vi "Configuration Tool Main.vi"() -> ()   [LabVIEW 2015, in "Configuration Tool.lvlib"]
doc: "This is the main VI for the configuration editor."
uses:
  Configuration Tool.lvlib
  Controls/StateCluster.ctl
  <vilib>/NI/Configuration Framework/Repository/NISE_CEF_Repository.lvclass
  <vilib>/NI/Configuration Framework/Node/NodeRef.ctl
  <vilib>/NI/Configuration Framework/Node/NISE_CEF_Node.lvclass
  <vilib>/NI/Configuration Framework/Node/StandardEvents.ctl
  <vilib>/NI/Configuration Framework/Node/UserEventRef.ctl
  <vilib>/NI/Configuration Framework/Controls/EventCluster.ctl
  <vilib>/NI/Configuration Framework/Node/NodeChangeEvent.ctl
  <vilib>/NI/Configuration Framework/Node/CacheState.ctl
  <vilib>/NI/Configuration Framework/Node/RefreshUIEvent.ctl
  <vilib>/NI/Configuration Framework/Node/StopEvent.ctl
  <vilib>/NI/Configuration Framework/glyph manager/glyph manager.ctl
  <vilib>/picture/picture.llb/imagedata.ctl
  Controls/AddMessage.ctl
  Controls/MoveMessage.ctl
  <vilib>/Utility/error.llb/DialogType.ctl
  Classes/cRIO/cRIO.lvclass
  Classes/cRIO Repo/cRIORepo.lvclass
  <vilib>/Utility/sysdir.llb/System Directory Type.ctl
  <vilib>/NI/AMC/Read Termination Message.vi
  <vilib>/NI/AMC/Create Single Message.vi
  <vilib>/NI/AMC/Update Message Routing Info.vi
  <vilib>/NI/AMC/Send Message.vi
  <vilib>/NI/AMC/Globals.vi
  <vilib>/NI/AMC/AMC.lvlib
  <vilib>/NI/Configuration Framework/NISE_CEF_TreeControl.lvlib
  <vilib>/NI/Configuration Framework/glyph manager/glyph manager.lvlib
panel:
  in  "View":string(tree)
  in  "Exit":bool
  # "Configurator"
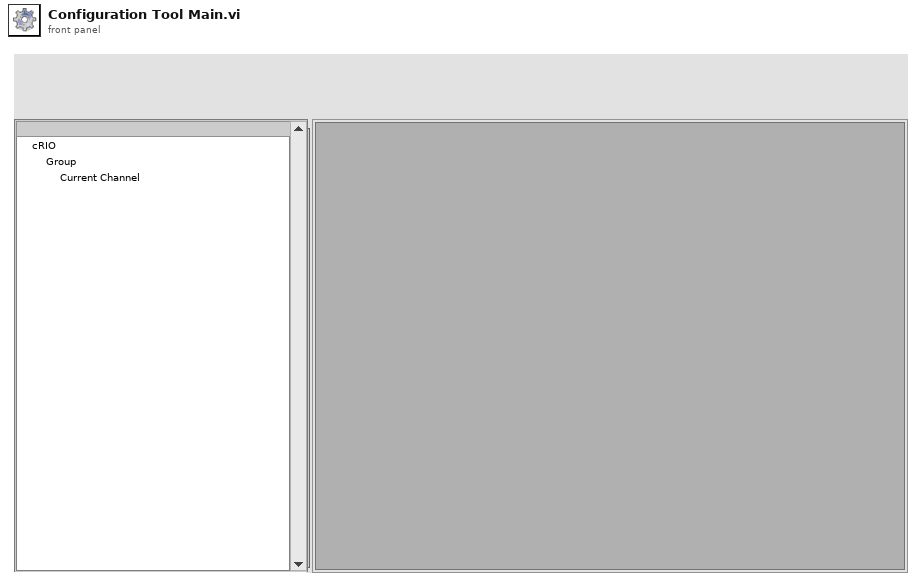
[diagram p1: front panel]
types:
  T1 = typedef "Configuration Tool.lvlib/StateCluster.ctl" = cluster{"repository":refnum<class "NISE_CEF_Repository.lvclass">, "root":T2, "unsaved changes":bool, "current path":path, "standard events":T3, "classes path":path, "glyph manager":T9}
  T2 = typedef "NISE_CEF_Node.lvclass/NodeRef.ctl" = refnum<data-value>
  T3 = typedef "NISE_CEF_Node.lvclass/StandardEvents.ctl" = cluster{"user event":T4, "node change":T5, "cache state":T6, "refresh UI":T7, "stop event":T8}
  T4 = typedef "NISE_CEF_Node.lvclass/UserEventRef.ctl" = refnum<user-event>
  T5 = typedef "NISE_CEF_Node.lvclass/NodeChangeEvent.ctl" = refnum<user-event>
  T6 = typedef "NISE_CEF_Node.lvclass/CacheState.ctl" = refnum<user-event>
  T7 = typedef "NISE_CEF_Node.lvclass/RefreshUIEvent.ctl" = refnum<user-event>
  T8 = typedef "NISE_CEF_Node.lvclass/StopEvent.ctl" = refnum<user-event>
  T9 = typedef "glyph manager.lvlib/glyph manager.ctl" = cluster{"search paths":path[], "glyph map":variant, "base glyphs":T10[], "desired overlays":string[]}
  T10 = typedef "imagedata.ctl" = cluster{"image type":i32, "image depth":i32, "image":u8[], "mask":u8[], "colors":u32[], "Rectangle":cluster{"left":i16, "top":i16, "right":i16, "bottom":i16}}
  T11 = typedef "AMC.lvlib/Message Queue.ctl" = refnum<queue>
  T12 = typedef "Configuration Tool.lvlib/AddMessage.ctl" = cluster{"node type":string, "to add to":string}
  T13 = typedef "Configuration Tool.lvlib/MoveMessage.ctl" = cluster{"node ref":T2, "new parent":T2}
  T14 = typedef "Configuration Tool.lvlib/FilePaths.ctl" = cluster{"glyphs":path, "classes":path}
  T15 = typedef "DialogType.ctl" = u16
  T16 = typedef "System Directory Type.ctl" = i32
  T17 = typedef "NISE_CEF_Node.lvclass/Summary.ctl" = cluster{"ID":string, "parent ID":string, "node type":string, "text":string, "additional text":string, "glyph":string, "depth":i32, "glyph overlay":string}
  T18 = typedef "LVPoint32TypeDef.ctl" = cluster{"Horizontal":i32, "Vertical":i32}
  T19 = cluster{"data name":string, "drag data":variant}[]
  T20 = typedef "NISE_CEF_Node.lvclass/NodeMenuOptions.ctl" = cluster{"removable":bool, "movable":bool, "duplicate":bool}
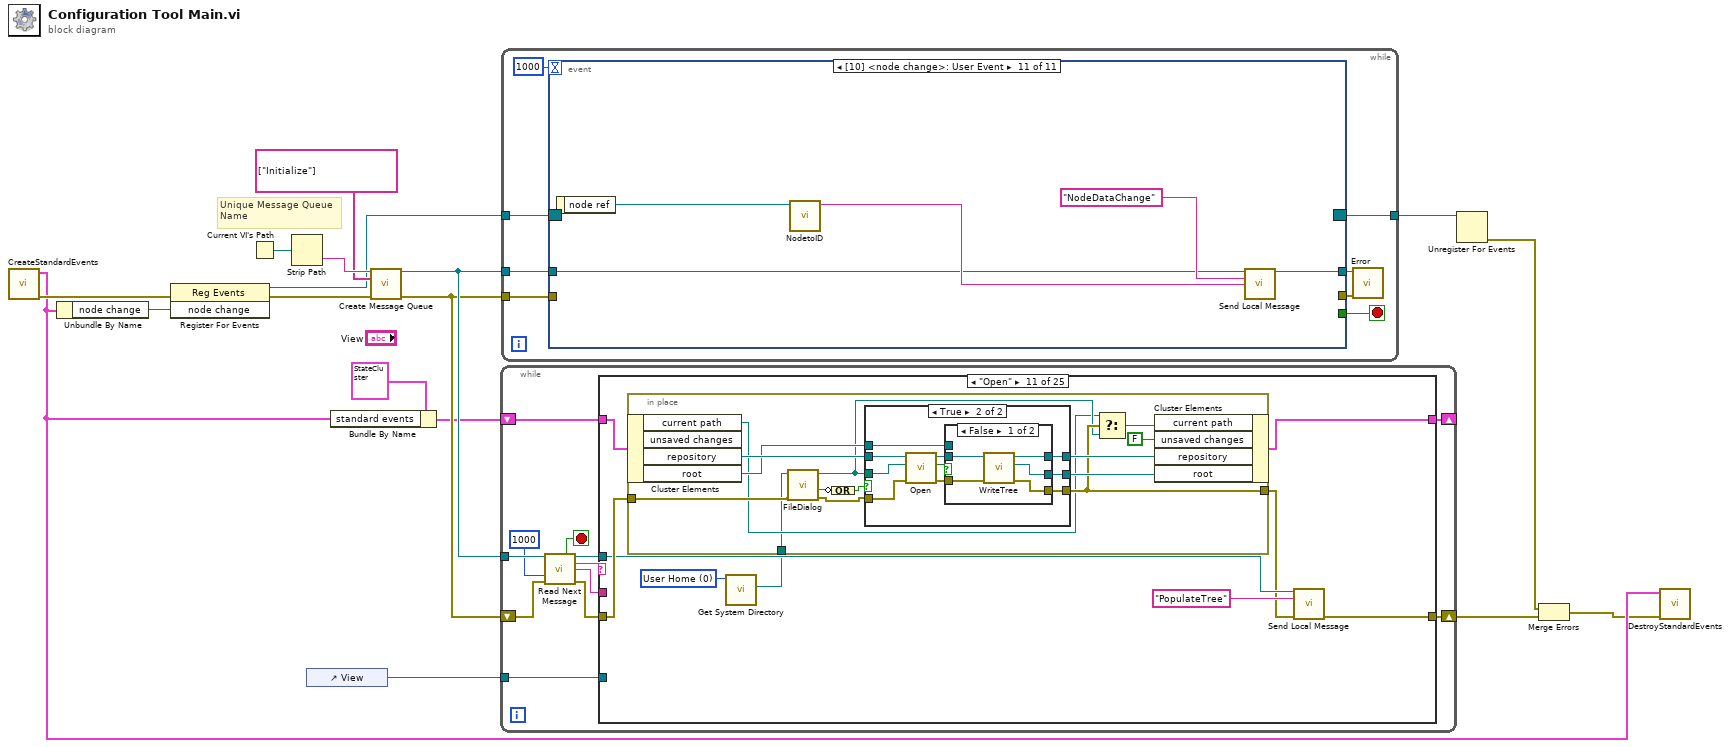
[diagram p0: block diagram]
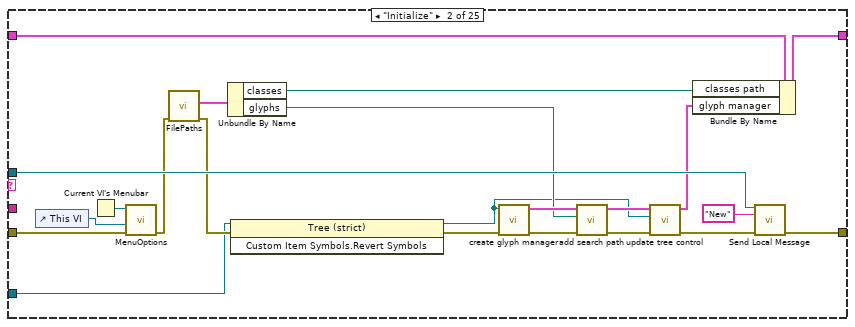
[diagram p3: hidden frame]
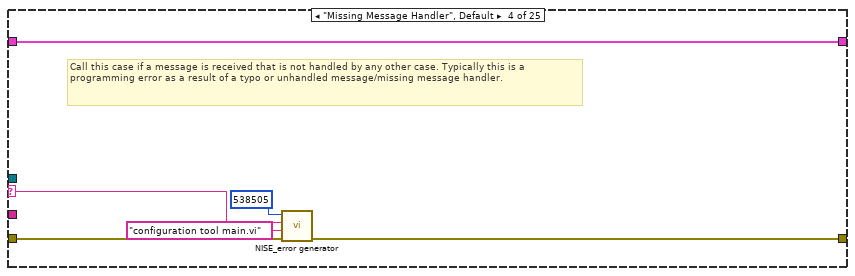
[diagram p5: hidden frame]
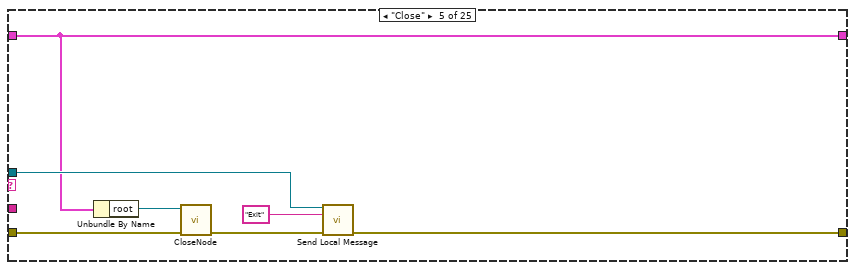
[diagram p6: hidden frame]
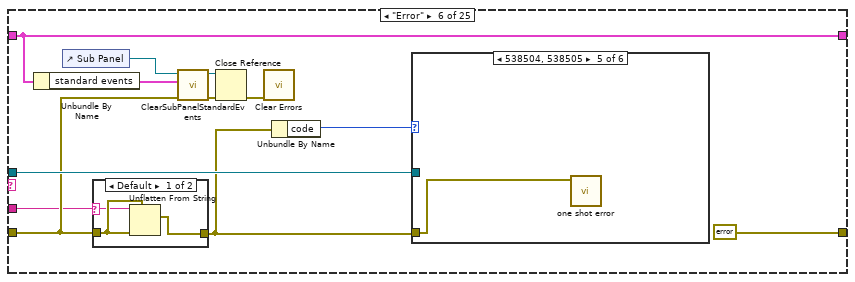
[diagram p7: hidden frame]
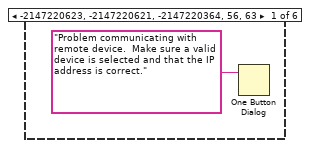
[diagram p9: hidden frame]
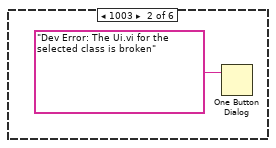
[diagram p10: hidden frame]
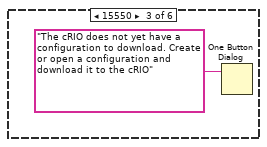
[diagram p11: hidden frame]
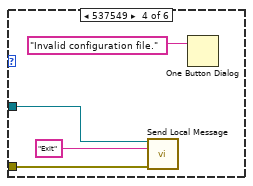
[diagram p12: hidden frame]
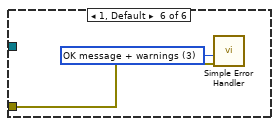
[diagram p13: hidden frame]
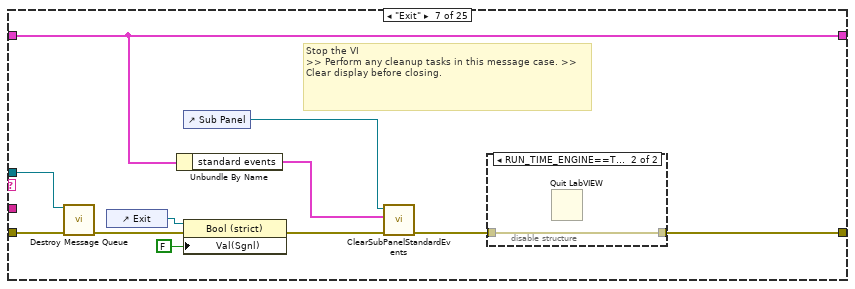
[diagram p14: hidden frame]
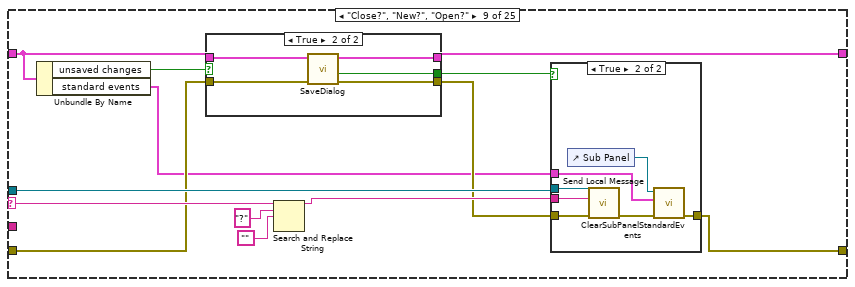
[diagram p17: hidden frame]
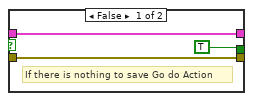
[diagram p18: hidden frame]
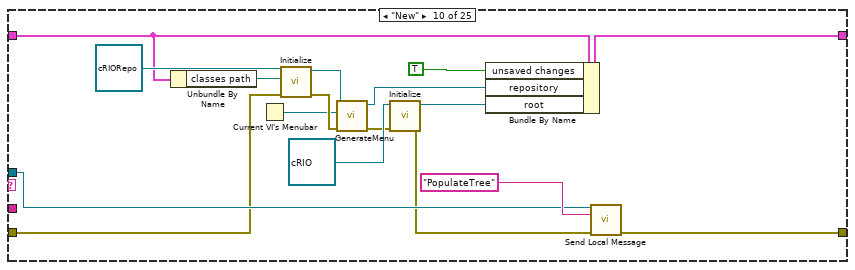
[diagram p20: hidden frame]
diagram:
  # "Unique Message Queue Name"
  n1 = call <vilib>:"CreateStandardEvents.vi"() -> ("error out"=w12:errorcluster, "standard events"=w6:T3)  [unwired: 10 in]
  n2 = Unbundle By Name(w6) -> ("node change"=w11:T5)
  n3 = register-events(error in=w12, w11) -> (reference out=w5:refnum<event-registration>, error out=w10:errorcluster)  [unwired: 1 in]
  n4 = Current VI's Path() -> (path=w16:path)
  n5 = Strip Path(path=w16) -> (name=w17:string)  [unwired: 1 out]
  n6 = control-ref of="View"() -> (w4:refnum<vi>)
  n7 = Bundle By Name(cluster=T1 {"repository"=refnum, "root"=refnum, "unsaved changes"=FALSE, "current path"=path "", "standard events"={"user event"=refnum, "node change"=refnum, "cache state"=refnum, "refresh UI"=refnum, "stop event"=refnum}, "classes path"=path "", "glyph manager"={"search paths"=[], "glyph map"=variant, "base glyphs"=[], "desired overlays"=[]}}, "standard events"=w6) -> (w8:T1)
  n8 = call <vilib>:"Create Message Queue.vi"("message queue name"=w17, "initial message names"=string[] ["Initialize"], "error in"=w10) -> ("message queue out"=w14:T11, "error out"=w13:errorcluster)  [unwired: 11 in]
  n9 = while "Message Processor" {
    shift-right: [w25] -> w7
    shift-left: w13 -> [w24]
    tunnel: w14 -> [w23]
    shift-right: [w21] -> _
    shift-left: w8 -> [w20]
    tunnel: w4 -> [w18]
    stop <- w29 stop-if-true
    n10 = call <vilib>:"Read Next Message.vi"("message queue in"=w23, "timeout (1 ms)"=1000, "error in"=w24) -> ("exit process?"=w29:bool, "message queue out"=w19:T11, "message name"=w28:string, "message value"=w27:string, "error out"=w26:errorcluster)  [unwired: 5 in, 3 out]
    n11 = case shown="\"Open\"" w28 {
      selector: w28 -> [_ _ _ w57 _ _ _ _ w118 _ _ _ _ _ _ _ _ w318 _ _ _ _ _ _ _]
      tunnel: w27 -> [_ _ _ _ _ w70 _ _ _ _ _ _ _ w236 _ w279 w296 w316 w368 w392 _ _ w432 w452 w459]
      tunnel: w26 -> [w31 w53 w55 w60 w63 w73 w105 w109 w111 w144 w162 w202 w228 w243 w256 w271 w295 w321 w370 w391 w413 w422 w431 w450 w460]
      tunnel: [w31 w49 w55 w58 w67 errorcluster {"status"=FALSE, "code"=0, "source"=""} ("error out") w97 w109 w122 w154 w158 w206 w230 w240 w256 w273 w299 w324 w372 w388 w407 w418 w428 w445 w458] -> w25
      tunnel: [w30 w45 w54 w61 w65 w77 w96 w108 w113 w152 w163 w209 w229 w237 w255 w265 w292 w325 w371 w393 w404 w421 w426 w453 w455] -> w21
      tunnel: w20 -> [w30 w46 w54 w61 w65 w77 w96 w108 w114 w147 w164 w204 w227 w238 w255 w269 w293 w325 w363 w393 w416 w421 w426 w453 w461]
      tunnel: w19 -> [_ w48 _ _ w66 w80 w104 _ w121 w153 w160 w205 _ w239 _ _ _ w319 _ _ _ _ w427 w444 w457]
      tunnel: w18 -> [_ w32 _ _ _ _ _ _ _ _ _ _ _ _ _ w266 w288 w313 w365 w386 w405 _ _ _ _]
      frame "------------Generic Operations------------" {
        # "Dummy case to add a seperation in the Case Structure menu"
      }
      frame "Initialize" {
        n12 = control-ref of="This VI"() -> (w52:refnum<vi>)
        n13 = Current VI's Menubar() -> (w51:refnum<k9>)
        n14 = call "MenuOptions.vi"("error in"=w53, "VI ref"=w52, "menu ref in"=w51) -> ("error out"=w44:errorcluster)  [unwired: 7 in, 1 out]
        n15 = call "FilePaths.vi"("error in"=w44) -> ("error out"=w35:errorcluster, "paths"=w47:T14)  [unwired: 9 in]
        n16 = Unbundle By Name(w47) -> ("classes"=w43:path, "glyphs"=w37:path)
        n17 = invoke class="Tree (strict)" method="Custom Item Symbols.Revert Symbols"(reference=w32, error in=w35) -> (reference out=w33:refnum<vi>, error out=w34:errorcluster)  [unwired: 1 in, 1 out]
        n18 = call <vilib>:"create glyph manager.vi"("error in"=w34, "tree ref (for default symbols)"=w33) -> ("error out"=w42:errorcluster, "glyph manager"=w41:T9)  [unwired: 8 in]
        n19 = call <vilib>:"add search path.vi"("error in"=w42, "search path"=w37, "glyph manager in"=w41) -> ("error out"=w40:errorcluster, "glyph manager out"=w39:T9)  [unwired: 7 in]
        n20 = call <vilib>:"update tree control.vi"("error in"=w40, "tree reference"=w33, "glyph manager in"=w39) -> ("error out"=w38:errorcluster, "glyph manager out"=w36:T9)  [unwired: 7 in]
        n21 = Bundle By Name(cluster=w46, "classes path"=w43, "glyph manager"=w36) -> (w45:T1)
        n22 = call <vilib>:"Send Local Message.vi"("message queue in"=w48, "message name"="New" ("Message Name"), "error in"=w38) -> ("error out"=w49:errorcluster)  [unwired: 10 in, 2 out]
      }
      frame "", "Idle" {
      }
      frame "Missing Message Handler", Default {
        # "Call this case if a message is received that is not handled by any other case. Typically this is a programming error as a result of a typo or unhandled message/missing message handler."
        n23 = call <vilib>:"NISE_error generator.vi"("error in"=w60, "source"="configuration tool main.vi", "append error message"=w57, "error code (0)"=538505) -> ("error out"=w58:errorcluster)  [unwired: 5 in]
      }
      frame "Close" {
        n24 = Unbundle By Name(w65) -> ("root"=w64:T2)
        n25 = call <vilib>:"CloseNode.vi"("error in"=w63, "node ref"=w64) -> ("error out"=w62:errorcluster)  [unwired: 9 in]
        n26 = call <vilib>:"Send Local Message.vi"("message queue in"=w66, "message name"="Exit", "error in"=w62) -> ("error out"=w67:errorcluster)  [unwired: 10 in, 2 out]
      }
      frame "Error" {
        n27 = Unbundle By Name(w77) -> ("standard events"=w69:T3)
        n28 = control-ref of="Sub Panel"() -> (w76:refnum<vi>)
        n29 = case shown="Default" w70 {
          selector: w70 -> [w82 _]
          tunnel: w73 -> [w83 w84]
          tunnel: [w81 w84] -> w72
          frame Default {
            n30 = Unflatten From String(type=w83, binary string=w82, error in (no error)=w83) -> (value=w81:errorcluster)  [unwired: 2 in, 2 out]
          }
          frame "" {
          }
        }
        n31 = call <vilib>:"ClearSubPanelStandardEvents.vi"("error in"=w73, "standard events"=w69, "sub panel ref in"=w76) -> ("error out"=w75:errorcluster, "sub panel ref out"=w74:refnum<vi>)  [unwired: 7 in]
        n32 = Close Reference(reference=w74, error in (no error)=w75) -> (error out=w71:errorcluster)
        n33 = call <vilib>:"Clear Errors.vi"("error in (no error)"=w71) -> ()  [unwired: 5 in, 2 out]
        n34 = Unbundle By Name(w72) -> ("code"=w78:i32)
        n35 = case shown="538504, 538505" w78 {
          tunnel: w80 -> [_ _ _ w90 _ _]
          tunnel: w72 -> [_ _ _ w89 w92 w94]
          frame -2147220623, -2147220621, -2147220364, 56, 63 {
            n36 = One Button Dialog(message="Problem communicating with remote device.  Make sure a valid device is selected and that the IP address is correct.") -> ()  [unwired: 1 in, 1 out]
          }
          frame 1003 {
            n37 = One Button Dialog(message="Dev Error: The Ui.vi for the selected class is broken") -> ()  [unwired: 1 in, 1 out]
          }
          frame 15550 {
            n38 = One Button Dialog(message="The cRIO does not yet have a configuration to download. Create or open a configuration and download it to the cRIO") -> ()  [unwired: 1 in, 1 out]
          }
          frame 537549 {
            n39 = call <vilib>:"Send Local Message.vi"("message queue in"=w90, "message name"="Exit", "error in"=w89) -> ()  [unwired: 10 in, 3 out]
            n40 = One Button Dialog(message="Invalid configuration file.") -> ()  [unwired: 1 in, 1 out]
          }
          frame 538504, 538505 {
            n41 = call <vilib>:"one shot error.vi"("error in"=w92) -> ()  [unwired: 11 in]
          }
          frame 1, Default {
            w93 = T15 3 items=["no dialog", "OK message", "continue or stop message", "OK message + warnings", "continue/stop + warnings"] ("type of dialog (OK msg:1)")
            n42 = call <vilib>:"Simple Error Handler.vi"("type of dialog (OK msg:1)"=w93, "error in (no error)"=w94) -> ()  [unwired: 8 out]
          }
        }
      }
      frame "Exit" {
        # "Stop the VI                                                                             >> Perform any cleanup tasks in this message case. >> Clear display before closing."
        n43 = call <vilib>:"Destroy Message Queue.vi"("message queue in"=w104, "error in"=w105) -> ("error out"=w101:errorcluster)  [unwired: 11 in, 2 out]
        n44 = control-ref of="Exit"() -> (w103:refnum<vi>)
        n45 = Unbundle By Name(w96) -> ("standard events"=w95:T3)
        n46 = control-ref of="Sub Panel"() -> (w100:refnum<vi>)
        n47 = property class="Bool (strict)"(reference=w103, error in=w101, "Val(Sgnl)"=FALSE ("Exit")) -> (error out=w99:errorcluster)  [unwired: 1 out]
        n48 = call <vilib>:"ClearSubPanelStandardEvents.vi"("error in"=w99, "standard events"=w95, "sub panel ref in"=w100) -> ("error out"=w98:errorcluster)  [unwired: 7 in, 1 out]
        n49 = disable-structure shown="RUN_TIME_ENGINE==True" {
          disable-tunnel: [w106 w107] -> w97
          disable-tunnel: w98 -> [w106 w107]
          frame condition #0 (active) {
          }
          frame condition #1 {
            n50 = Quit LabVIEW() -> ()  [unwired: 1 in]
          }
        }
      }
      frame "------------Menu Operations--------------" {
        # "Dummy case to add a seperation in the Case Structure menu"
      }
      frame "Close?", "New?", "Open?" {
        n51 = Unbundle By Name(w114) -> ("unsaved changes"=w116:bool, "standard events"=w110:T3)
        n52 = case shown="True" w116 {
          tunnel: [TRUE ("SaveFlag") w130] -> w115
          tunnel: w114 -> [w124 w129]
          tunnel: [w124 w128] -> w113
          tunnel: w111 -> [w123 w127]
          tunnel: [w123 w126] -> w112
          frame False {
            # "If there is nothing to save Go do Action"
          }
          frame True {
            n53 = call "SaveDialog.vi"("error in"=w127, "state in"=w129) -> ("error out"=w126:errorcluster, "new"=w130:bool, "state out"=w128:T1)  [unwired: 7 in]
          }
        }
        n54 = Search and Replace String(input string=w118, search string="?", replace string="") -> (result string=w117:string)  [unwired: 5 in, 3 out]
        n55 = case shown="True" w115 {
          tunnel: w112 -> [w131 w138]
          tunnel: [w131 w134] -> w122
          tunnel: w121 -> [_ w137]
          tunnel: w117 -> [_ w136]
          tunnel: w110 -> [_ w132]
          frame False {
          }
          frame True {
            n56 = control-ref of="Sub Panel"() -> (w133:refnum<vi>)
            n57 = call <vilib>:"Send Local Message.vi"("message queue in"=w137, "message name"=w136, "error in"=w138) -> ("error out"=w135:errorcluster)  [unwired: 10 in, 2 out]
            n58 = call <vilib>:"ClearSubPanelStandardEvents.vi"("error in"=w135, "standard events"=w132, "sub panel ref in"=w133) -> ("error out"=w134:errorcluster)  [unwired: 7 in, 1 out]
          }
        }
      }
      frame "New" {
        n59 = Unbundle By Name(w147) -> ("classes path"=w146:path)
        n60 = Current VI's Menubar() -> (w139:refnum<k9>)
        n61 = call-dynamic "Initialize.vi"("error in"=w144, "path"=w146, "repository in"=refnum<class "cRIORepo.lvclass"> refnum ("cRIORepo.lvclass")) -> ("error out"=w143:errorcluster, "repository out"=w141:refnum<class "cRIORepo.lvclass">)  [unwired: 7 in]
        n62 = call-dynamic "GenerateMenu.vi"("error in"=w143, "menu ref in"=w139, "NISE_CEF_Repository in"=w141) -> ("error out"=w142:errorcluster, "NISE_CEF_Repository out"=w140:refnum<class "cRIORepo.lvclass">)  [unwired: 6 in, 1 out]
        n63 = call-dynamic "Initialize.vi"("error in"=w142, "cRIO in"=refnum<class "cRIO.lvclass"> refnum ("cRIO.lvclass")) -> ("error out"=w145:errorcluster, "data value reference"=w149:T2)  [unwired: 7 in, 1 out]
        n64 = Bundle By Name(cluster=w147, "unsaved changes"=TRUE ("SaveFlag"), "repository"=w140, "root"=w149) -> (w152:T1)
        n65 = call <vilib>:"Send Local Message.vi"("message queue in"=w153, "message name"="PopulateTree", "error in"=w145) -> ("error out"=w154:errorcluster)  [unwired: 10 in, 2 out]
      }
      frame "Open" {
        w157 = T16 0 items=["User Home"=0, "User Desktop"=1, "User Documents"=2, "User Application Data"=3, "User Preferences"=4, "User Temporary"=5, "Public Documents"=6, "Public Application Data"=7, "Public Preferences"=8, "Public Cache"=13, "System Core Libraries"=9, "System Installed Libraries"=10, "Application Files"=11, "Boot Volume Root"=12] ("system directory type")
        n66 = call <vilib>:"Get System Directory.vi"("system directory type"=w157) -> ("system directory"=w156:path)  [unwired: 10 in]
        n67 = in-place {
          in-place-border: w162 -> [w170]
          in-place-border: [w169] -> w159
          in-place-border: w156 -> [w165]
          n68 = in-place-cluster #1(w164) -> ("current path"=w167:path, "repository"=w178:refnum<class "NISE_CEF_Repository.lvclass">, "root"=w174:T2)  [unwired: 1 out]
          n69 = call "FileDialog.vi"("error in"=w170, "start path"=w165) -> ("error out"=w171:errorcluster, "cancelled"=w172:bool, "selected path"=w168:path)  [unwired: 7 in]
          n70 = Compound Arithmetic op=OR(invert w172) -> (w173:bool)
          n71 = case shown="True" w173 {
            tunnel: w178 -> [w179 w191]
            tunnel: [w179 w189] -> w176
            tunnel: [w180 w187] -> w169
            tunnel: [w181 w186] -> w175
            tunnel: w168 -> [_ w184]
            tunnel: w171 -> [w180 w183]
            tunnel: w174 -> [w181 w182]
            frame False {
            }
            frame True {
              n72 = call-dynamic "Open.vi"("error in"=w183, "file path"=w184, "repository in"=w191) -> ("error out"=w188:errorcluster, "invalid?"=w185:bool, "repository out"=w190:refnum<class "NISE_CEF_Repository.lvclass">)  [unwired: 6 in]
              n73 = case shown="False" w185 {
                tunnel: w190 -> [w196 w199]
                tunnel: [w195 w199] -> w189
                tunnel: w188 -> [w194 w198]
                tunnel: [w193 w198] -> w187
                tunnel: [w192 w197] -> w186
                tunnel: w182 -> [_ w197]
                frame False {
                  n74 = call-dynamic "WriteTree.vi"("error in"=w194, "repository in"=w196) -> ("error out"=w193:errorcluster, "root"=w192:T2, "repository out"=w195:refnum<class "NISE_CEF_Repository.lvclass">)  [unwired: 7 in]
                }
                frame True {
                }
              }
            }
          }
          n75 = Select(t=w167, s=w169, f=w168) -> (s? t:f=w166:path)
          n76 = in-place-cluster #1("current path"=w166, "unsaved changes"=FALSE ("SaveFlag"), "repository"=w176, "root"=w175) -> (w163:T1)
        }
        n77 = call <vilib>:"Send Local Message.vi"("message queue in"=w160, "message name"="PopulateTree", "error in"=w159) -> ("error out"=w158:errorcluster)  [unwired: 10 in, 2 out]
      }
      frame "Save" {
        n78 = in-place {
          in-place-border: w202 -> [w213]
          in-place-border: [w212] -> w201
          in-place-border: [w210] -> w200
          n79 = in-place-cluster #2(w204) -> ("current path"=w211:path, "root"=w214:T2, "repository"=w216:refnum<class "NISE_CEF_Repository.lvclass">)
          n80 = Empty String/Path?(string/path=w211) -> (empty?=w210:bool)
          n81 = call-dynamic "ReadTree.vi"("error in"=w213, "root"=w214, "repository in"=w216) -> ("error out"=w212:errorcluster, "repository out"=w215:refnum<class "NISE_CEF_Repository.lvclass">)  [unwired: 7 in]
          n82 = in-place-cluster #2("current path"=w211, "root"=w214, "repository"=w215) -> (w203:T1)
        }
        n83 = case shown="True" w200 {
          tunnel: w203 -> [w220 w222]
          tunnel: [w219 w221] -> w209
          tunnel: [w218 w223] -> w207
          tunnel: w201 -> [w217 w224]
          frame False {
            n84 = call "Save.vi"("error in"=w217, "state in"=w220) -> ("error out"=w218:errorcluster, "state out"=w219:T1)  [unwired: 8 in]
          }
          frame True {
            # "Empty path use Dialog"
            n85 = call "SaveAs.vi"("error in"=w224, "state in"=w222) -> ("error out"=w223:errorcluster, "state out"=w221:T1)  [unwired: 7 in, 1 out]
          }
        }
        n86 = call <vilib>:"Send Local Message.vi"("message queue in"=w205, "message name"="PopulateTree", "error in"=w207) -> ("error out"=w206:errorcluster)  [unwired: 10 in, 2 out]
      }
      frame "SaveAs" {
        n87 = in-place {
          in-place-border: w228 -> [w232]
          in-place-border: [w231] -> w226
          n88 = in-place-cluster #3(w227) -> ("root"=w233:T2, "repository"=w235:refnum<class "NISE_CEF_Repository.lvclass">)
          n89 = call-dynamic "ReadTree.vi"("error in"=w232, "root"=w233, "repository in"=w235) -> ("error out"=w231:errorcluster, "repository out"=w234:refnum<class "NISE_CEF_Repository.lvclass">)  [unwired: 7 in]
          n90 = in-place-cluster #3("root"=w233, "repository"=w234) -> (w225:T1)
        }
        n91 = call "SaveAs.vi"("error in"=w226, "state in"=w225) -> ("error out"=w230:errorcluster, "state out"=w229:T1)  [unwired: 7 in, 1 out]
      }
      frame "Custom View" {
        n92 = in-place {
          in-place-border: w243 -> [w254]
          in-place-border: [w253] -> w241
          in-place-border: w236 -> [w244]
          n93 = in-place-cluster #4(w238) -> ("repository"=w248:refnum<class "NISE_CEF_Repository.lvclass">, "root"=w247:T2)
          n94 = call-dynamic "ReadTree.vi"("error in"=w254, "root"=w247, "repository in"=w248) -> ("error out"=w251:errorcluster, "repository out"=w250:refnum<class "NISE_CEF_Repository.lvclass">)  [unwired: 7 in]
          n95 = call-dynamic "CustomView.vi"("error in"=w251, "view name"=w244, "repository in"=w250) -> ("error out"=w252:errorcluster, "repository out"=w249:refnum<class "NISE_CEF_Repository.lvclass">)  [unwired: 7 in]
          n96 = call-dynamic "WriteTree.vi"("error in"=w252, "repository in"=w249) -> ("error out"=w253:errorcluster, "root"=w245:T2, "repository out"=w246:refnum<class "NISE_CEF_Repository.lvclass">)  [unwired: 7 in]
          n97 = in-place-cluster #4("repository"=w246, "root"=w245) -> (w237:T1)
        }
        n98 = call <vilib>:"Send Local Message.vi"("message queue in"=w239, "message name"="PopulateTree", "error in"=w241) -> ("error out"=w240:errorcluster)  [unwired: 10 in, 2 out]
      }
      frame "-------TreeControl Operations-----------" {
        # "Dummy case to add a seperation in the Case Structure menu"
      }
      frame "AddNode" {
        n99 = Unflatten From String(type=T12 {"node type"="", "to add to"=""} ("input cluster"), binary string=w279) -> (value=w277:T12)  [unwired: 3 in, 2 out]
        n100 = Unbundle By Name(w277) -> ("to add to"=w275:string, "node type"=w268:string)
        n101 = in-place {
          in-place-border: w271 -> [w285]
          in-place-border: [w284] -> w270
          in-place-border: w268 -> [w283]
          in-place-border: [w282] -> w267
          n102 = in-place-cluster #5(w269) -> ("repository"=w287:refnum<class "NISE_CEF_Repository.lvclass">)
          n103 = call-dynamic "GetClassPath.vi"("error in"=w285, "class name"=w283, "Repository in"=w287) -> ("error out"=w284:errorcluster, "class path"=w282:path, "Repository out"=w286:refnum<class "NISE_CEF_Repository.lvclass">)  [unwired: 6 in]
          n104 = in-place-cluster #5("repository"=w286) -> (w262:T1)
        }
        n105 = Unbundle By Name(w262) -> ("glyph manager"=w261:T9)
        n106 = call <vilib>:"Get LV Class Default Value.vi"("error in (no error)"=w270, "class path"=w267) -> ("error out"=w280:errorcluster, "object"=w281:refnum<class>)  [unwired: 8 in]
        n107 = To More Specific Class(target class=refnum<class "NISE_CEF_Node.lvclass"> refnum ("Node.lvclass"), reference=w281, error in=w280) -> (specific class reference=w263:refnum<class "NISE_CEF_Node.lvclass">, error out=w264:errorcluster)
        n108 = call-dynamic "AddGlyphtoGManager.vi"("error in"=w264, "glyph manager"=w261, "NISE_CEF_Node in"=w263) -> ("error out"=w259:errorcluster, "glyph manager out"=w260:T9, "NISE_CEF_Node out"=w258:refnum<class "NISE_CEF_Node.lvclass">)  [unwired: 6 in]
        n109 = call <vilib>:"AddNode.vi"("error in"=w259, "node in"=w258, "parent node ID"=w275) -> ("error out"=w274:errorcluster, "summary"=w272:T17[])  [unwired: 7 in]
        n110 = call <vilib>:"PopulateTreeSumaryWithGlyphManager.vi"("error in"=w274, "glyph manager"=w260, "summary"=w272, "tree ref in"=w266) -> ("error out"=w273:errorcluster, "glyph manager out"=w257:T9)  [unwired: 6 in]
        n111 = Bundle By Name(cluster=w262, "glyph manager"=w257) -> (w265:T1)
      }
      frame "Duplicate" {
        n112 = call <vilib>:"IDtoNode.vi"("error in"=w295, "ID"=w296) -> ("error out"=w297:errorcluster, "invalid Id"=w294:bool, "node ref"=w298:T2)  [unwired: 7 in]
        n113 = Unbundle By Name(w293) -> ("glyph manager"=w290:T9)
        n114 = case shown="False" w294 {
          tunnel: [w310 w312] -> w299
          tunnel: w298 -> [w309 _]
          tunnel: w297 -> [w306 w312]
          tunnel: w290 -> [w302 w311]
          tunnel: [w301 w311] -> w289
          tunnel: w288 -> [w300 _]
          frame False {
            n115 = call <vilib>:"DuplicateNode.vi"("same parent?"=TRUE ("s"), "error in"=w306, "node ref in"=w309) -> ("error out"=w307:errorcluster, "new node ref"=w308:T2)  [unwired: 7 in]
            n116 = call <vilib>:"Summary.vi"("error in"=w307, "node self ref"=w308) -> ("error out"=w304:errorcluster, "summary"=w303:T17[])  [unwired: 8 in]
            n117 = call <vilib>:"PopulateTreeSumaryWithGlyphManager.vi"("error in"=w304, "glyph manager"=w302, "summary"=w303, "tree ref in"=w300) -> ("error out"=w310:errorcluster, "glyph manager out"=w301:T9)  [unwired: 6 in]
          }
          frame True {
          }
        }
        n118 = Bundle By Name(cluster=w293, "unsaved changes"=TRUE, "glyph manager"=w289) -> (w292:T1)
      }
      frame "CustomMenuAction" {
        n119 = Match Pattern(string=w316, regular expression=":") -> (before substring=w315:string, after substring=w314:string)  [unwired: 1 in, 2 out]
        n120 = call <vilib>:"IDtoNode.vi"("error in"=w321, "ID"=w314) -> ("error out"=w322:errorcluster, "invalid Id"=w320:bool, "node ref"=w323:T2)  [unwired: 7 in]
        n121 = case shown="False" w320 {
          tunnel: [w331 w361] -> w324
          tunnel: w323 -> [w328 _]
          tunnel: w322 -> [w334 w361]
          tunnel: w319 -> [w335 _]
          tunnel: w318 -> [_ _]
          tunnel: w315 -> [w332 _]
          tunnel: w313 -> [w329 _]
          frame False {
            n122 = in-place {
              in-place-border: w335 -> [w359]
              in-place-border: w334 -> [w357]
              in-place-border: [w356] -> w330
              in-place-border: [w355] -> w333
              in-place-border: w332 -> [w354]
              in-place-border: w329 -> [w353]
              in-place-border: [w352] -> w327
              n123 = in-place-dvr #6(w328) -> (w360:refnum<class "NISE_CEF_Node.lvclass">)  [unwired: 1 out]
              n124 = call-dynamic "MenuHandler.vi"("tree control"=w353, "main message queue"=w359, "error in"=w357, "menu string"=w354, "NISE_CEF_Node in"=w360) -> ("error out"=w356:errorcluster, "refresh tree?"=w352:bool, "Unhandled"=w355:bool, "NISE_CEF_Node out"=w358:refnum<class "NISE_CEF_Node.lvclass">)  [unwired: 3 in]
              n125 = in-place-dvr #6(w358) -> (w326:T2)  [unwired: 1 out]
            }
            n126 = case shown="False" w333 {
              tunnel: w332 -> [_ w347]
              tunnel: [w339 w348] -> w331
              tunnel: w330 -> [w337 w349]
              tunnel: w327 -> [w336 _]
              tunnel: w326 -> [w338 _]
              frame False {
                n127 = case shown="False" w336 {
                  tunnel: [w340 w343] -> w339
                  tunnel: w338 -> [_ w342]
                  tunnel: w337 -> [w340 w341]
                  frame False {
                  }
                  frame True {
                    n128 = call <vilib>:"NodetoID.vi"("error in"=w341, "node ref"=w342) -> ("error out"=w345:errorcluster, "ID"=w346:string)  [unwired: 8 in]
                    n129 = call <vilib>:"Send Local Message.vi"("message name"="NodeDataChange", "message value"=w346, "error in"=w345) -> ("error out"=w343:errorcluster)  [unwired: 10 in, 2 out]
                  }
                }
              }
              frame True {
                n130 = call <vilib>:"NISE_error generator.vi"("error in"=w349, "source"="configuration tool main.vi", "append error message"=w347, "error code (0)"=538506) -> ("error out"=w348:errorcluster)  [unwired: 5 in]
              }
            }
          }
          frame True {
          }
        }
      }
      frame "RefreshNode" {
        # "Refreshes the node in the Tree, Sets the save flag to true. This case can be called from the UIs of the nodes"
        n131 = Unbundle By Name(w363) -> ("glyph manager"=w362:T9)
        n132 = call <vilib>:"IDtoNode.vi"("error in"=w370, "ID"=w368) -> ("error out"=w369:errorcluster, "invalid Id"=w366:bool, "node ref"=w367:T2)  [unwired: 7 in]
        n133 = case shown="False" w366 {
          tunnel: [w382 w385] -> w372
          tunnel: w369 -> [w378 w385]
          tunnel: w367 -> [w377 _]
          tunnel: w365 -> [w376 _]
          tunnel: [w375 w384] -> w364
          tunnel: w362 -> [w373 w384]
          frame False {
            n134 = call <vilib>:"SummaryWithGlyphManager.vi"("error in"=w378, "glyph manager"=w373, "node self ref"=w377) -> ("error out"=w380:errorcluster, "glyph manager out"=w374:T9, "summary"=w379:T17[])  [unwired: 6 in]
            n135 = call <vilib>:"RefreshSubTreeWithGlyphManager.vi"("error in"=w380, "glyph manager"=w374, "node information"=w379, "tree ref in"=w376) -> ("error out"=w383:errorcluster, "glyph manager out"=w375:T9, "tree ref out"=w381:refnum<vi>)  [unwired: 5 in]
            n136 = Close Reference(reference=w381, error in (no error)=w383) -> (error out=w382:errorcluster)
          }
          frame True {
          }
        }
        n137 = Bundle By Name(cluster=w363, "glyph manager"=w364) -> (w371:T1)
      }
      frame "RemoveNode" {
        n138 = call <vilib>:"IDtoNode.vi"("error in"=w391, "ID"=w392) -> ("error out"=w390:errorcluster, "invalid Id"=w387:bool, "node ref"=w389:T2)  [unwired: 7 in]
        n139 = case shown="False" w387 {
          tunnel: w390 -> [w399 w400]
          tunnel: w389 -> [w398 _]
          tunnel: [w395 w400] -> w388
          tunnel: w386 -> [w394 _]
          frame False {
            n140 = call <vilib>:"RemoveNode.vi"("error in"=w399, "node"=w398) -> ("error out"=w396:errorcluster, "node ID"=w397:string)  [unwired: 8 in]
            n141 = call <vilib>:"ClearTreeNode.vi"("error in"=w396, "tag"=w397, "tree reference"=w394) -> ("error out"=w395:errorcluster)  [unwired: 8 in]
          }
          frame True {
          }
        }
      }
      frame "PopulateTree" {
        n142 = Unbundle By Name(w416) -> ("standard events"=w406:T3, "glyph manager"=w402:T9, "root"=w411:T2)
        n143 = call <vilib>:"SummaryWithGlyphManager.vi"("error in"=w413, "glyph manager"=w402, "depth"=0 ("Depth"), "node self ref"=w411) -> ("error out"=w412:errorcluster, "glyph manager out"=w401:T9, "summary"=w415:T17[])  [unwired: 5 in]
        n144 = control-ref of="This VI"() -> (w414:refnum<vi>)
        n145 = call <vilib>:"RefreshEntireTreeWithGlyphManager.vi"("calling VI in"=w414, "error in"=w412, "glyph manager"=w401, "array"=w415, "tree ref in"=w405) -> ("error out"=w408:errorcluster, "glyph manager out"=w403:T9)  [unwired: 5 in]
        n146 = control-ref of="Sub Panel"() -> (w409:refnum<vi>)
        n147 = Bundle By Name(cluster=w416, "glyph manager"=w403) -> (w404:T1)
        n148 = call <vilib>:"ClearSubPanelStandardEvents.vi"("error in"=w408, "standard events"=w406, "sub panel ref in"=w409) -> ("error out"=w407:errorcluster)  [unwired: 7 in, 1 out]
      }
      frame "CleansubPanel" {
        n149 = Unbundle By Name(w421) -> ("standard events"=w417:T3)
        n150 = control-ref of="Sub Panel"() -> (w423:refnum<vi>)
        n151 = call <vilib>:"ClearSubPanelStandardEvents.vi"("error in"=w422, "standard events"=w417, "sub panel ref in"=w423) -> ("error out"=w420:errorcluster, "sub panel ref out"=w419:refnum<vi>)  [unwired: 7 in]
        n152 = Close Reference(reference=w419, error in (no error)=w420) -> (error out=w418:errorcluster)
      }
      frame "ActivateNode" {
        n153 = Unbundle By Name(w426) -> ("standard events"=w425:T3)
        n154 = call <vilib>:"IDtoNode.vi"("error in"=w431, "ID"=w432) -> ("error out"=w424:errorcluster, "invalid Id"=w430:bool, "node ref"=w429:T2)  [unwired: 7 in]
        n155 = case shown="False" w430 {
          tunnel: w429 -> [w439 _]
          tunnel: [w440 w441] -> w428
          tunnel: w424 -> [w437 w441]
          tunnel: w427 -> [w435 _]
          tunnel: w425 -> [w433 _]
          frame False {
            n156 = control-ref of="Sub Panel"() -> (w436:refnum<vi>)
            n157 = call <vilib>:"ClearSubPanelStandardEvents.vi"("error in"=w437, "standard events"=w433, "sub panel ref in"=w436) -> ("error out"=w438:errorcluster, "sub panel ref out"=w434:refnum<vi>)  [unwired: 7 in]
            n158 = call <vilib>:"LoadNodeUIStandardEvents.vi"("user event out"=w433, "error in"=w438, "sub panel ref in"=w434, "main queue"=w435, "node"=w439) -> ("error out"=w440:errorcluster)  [unwired: 6 in]
          }
          frame True {
          }
        }
      }
      frame "Move" {
        n159 = Unflatten From String(type=T13 {"node ref"=refnum, "new parent"=refnum} ("Cluster"), binary string=w452, error in (no error)=w450) -> (value=w449:T13, error out=w448:errorcluster)  [unwired: 2 in, 1 out]
        n160 = Unbundle By Name(w449) -> ("node ref"=w443:T2, "new parent"=w442:T2)
        n161 = call <vilib>:"MoveNode.vi"("error in"=w448, "new parent"=w442, "node"=w443) -> ("error out"=w446:errorcluster)  [unwired: 8 in]
        n162 = call <vilib>:"Send Local Message.vi"("message queue in"=w444, "message name"="PopulateTree", "error in"=w446) -> ("error out"=w445:errorcluster)  [unwired: 10 in, 2 out]
      }
      frame "NodeDataChange" {
        n163 = call <vilib>:"Send Local Message.vi"("message queue in"=w457, "message name"="RefreshNode", "message value"=w459, "error in"=w460) -> ("error out"=w458:errorcluster)  [unwired: 9 in, 2 out]
        n164 = Bundle By Name(cluster=w461, "unsaved changes"=TRUE) -> (w455:T1)
      }
    }
  }
  n165 = while "User Interface Event Handler" {
    tunnel: w14 -> [w468]
    tunnel: w13 -> [w464]
    tunnel: w5 -> [w463]
    tunnel: [w462] -> w1
    stop <- w467 stop-if-true
    n166 = event shown="[10] <node change>: User Event" {
      selector: w463 -> [_ _ _ _ _ _ _ _ _ _ _]
      dyn-events: [_ _ _ _ _ _ _ _ _ _ _] -> w462
      timeout: 1000 -> [_ _ _ _ _ _ _ _ _ _ _]
      tunnel: w468 -> [w471 w479 w503 w555 w583 w590 w619 w623 w633 w639 w685]
      tunnel: [_ _ _ _ TRUE _ _ _ _ _ _] -> w467
      tunnel: [w471 w479 w500 w553 w579 w590 w616 w623 w631 w638 w686] -> w466
      tunnel: [w470 w475 w499 w552 w580 w586 w615 w620 w629 w636 _] -> w465
      tunnel: w464 -> [w470 w478 w498 w554 w581 w589 w614 w622 w630 w637 _]
      event Timeout {
        # "Timeout code can be added here for autosave or Lock Screen"
        n167 = event-data() -> ()  [unwired: 1 in, 1 out]
      }
      event "View": Shortcut Menu Activation? {
        n168 = event-data() -> ("CtlRef"=w485:refnum<vi>, "Coords"=w484:T18, "MenuRef"=w481:refnum<k9>)  [unwired: 1 in]
        n169 = invoke class="Tree (strict)" method="Point To Row Column"(reference=w485, error in=w478, "Point"=w484) -> (error out=w477:errorcluster, "Tag"=w483:string)  [unwired: 5 in, 6 out]
        n170 = call <vilib>:"IDtoNode.vi"("error in"=w477, "ID"=w483) -> ("error out"=w473:errorcluster, "invalid Id"=w480:bool, "node ref"=w482:T2)  [unwired: 7 in]
        n171 = case shown="False" w480 {
          tunnel: w482 -> [w490 _]
          tunnel: w481 -> [w489 _]
          tunnel: [w488 _] -> w476
          tunnel: [w487 _] -> w474
          tunnel: w473 -> [w486 w496]
          tunnel: [w486 w496] -> w472
          frame False {
            n172 = in-place {
              in-place-border: w489 -> [w493]
              in-place-border: [w491] -> w488
              n173 = in-place-dvr #7(w490) -> (w495:refnum<class "NISE_CEF_Node.lvclass">, w492:errorcluster)
              n174 = call-dynamic "ShortcutMenu.vi"("error in"=w492, "menu ref in"=w493, "node in"=w495) -> ("error out"=w491:errorcluster, "node out"=w494:refnum<class "NISE_CEF_Node.lvclass">)  [unwired: 6 in, 1 out]
              n175 = in-place-dvr #7(w494) -> (w487:errorcluster)  [unwired: 1 out]
            }
          }
          frame True {
          }
        }
        n176 = Merge Errors(w474, w476, w472) -> (w475:errorcluster)
        n177 = event-data() -> ()  [unwired: 2 in, 1 out]
      }
      event "View": Shortcut Menu Selection (User) {
        n178 = event-data() -> ("ItemPath"=w502:string, "CtlRef"=w506:refnum<vi>, "Coords"=w507:T18)  [unwired: 1 in]
        n179 = invoke class="Tree (strict)" method="Point To Row Column"(reference=w506, error in=w498, "Point"=w507) -> (error out=w497:errorcluster, "Tag"=w501:string)  [unwired: 5 in, 6 out]
        n180 = Match Pattern(string=w502, regular expression=":") -> (before substring=w505:string, after substring=w504:string)  [unwired: 1 in, 2 out]
        n181 = case shown="Default" w505 {
          selector: w505 -> [w509 _ _ _]
          tunnel: w504 -> [_ _ _ w534]
          tunnel: w503 -> [w516 w523 w529 w536]
          tunnel: w501 -> [w511 w521 w527 w535]
          tunnel: [w513 w520 w526 w532] -> w500
          tunnel: [w514 w519 w524 w530] -> w499
          tunnel: w497 -> [w515 w518 w525 w531]
          frame Default {
            n182 = Concatenate Strings(w509, ":" ("string"), w511) -> (w512:string)
            n183 = call <vilib>:"Send Local Message.vi"("message queue in"=w516, "message name"="CustomMenuAction" ("Message Name"), "message value"=w512, "error in"=w515) -> ("message queue out"=w513:T11, "error out"=w514:errorcluster)  [unwired: 9 in, 1 out]
          }
          frame "Remove" {
            n184 = call <vilib>:"Send Local Message.vi"("message queue in"=w523, "message name"="RemoveNode" ("Message Name"), "message value"=w521, "error in"=w518) -> ("message queue out"=w520:T11, "error out"=w519:errorcluster)  [unwired: 9 in, 1 out]
          }
          frame "Duplicate" {
            n185 = call <vilib>:"Send Local Message.vi"("message queue in"=w529, "message name"="Duplicate" ("Message Name"), "message value"=w527, "error in"=w525) -> ("message queue out"=w526:T11, "error out"=w524:errorcluster)  [unwired: 9 in, 1 out]
          }
          frame "Add" {
            n186 = Bundle By Name(cluster=T12 {"node type"="", "to add to"=""} ("input cluster"), "node type"=w534, "to add to"=w535) -> (w537:T12)
            n187 = Flatten To String(anything=w537) -> (data string=w538:string)  [unwired: 3 in, 2 out]
            n188 = call <vilib>:"Send Local Message.vi"("message queue in"=w536, "message name"="AddNode" ("Message Name"), "message value"=w538, "error in"=w531) -> ("message queue out"=w532:T11, "error out"=w530:errorcluster)  [unwired: 9 in, 1 out]
          }
        }
      }
      event "View": Drop {
        n189 = event-data() -> ("CtlRef"=w558:refnum<vi>, "Coords"=w557:T18)  [unwired: 1 in]
        n190 = invoke class="Tree (strict)" method="Point To Row Column"(reference=w558, error in=w554, "Point"=w557) -> (reference out=w556:refnum<vi>, error out=w551:errorcluster, "Tag"=w548:string)  [unwired: 5 in, 5 out]
        n191 = call <vilib>:"ValidDragDrop.vi"("error in"=w551, "drag over"=w548, "tree ref in"=w556) -> ("error out"=w543:errorcluster, "accepted"=w546:bool, "drag"=w550:string, "tree ref out"=w560:refnum<vi>)  [unwired: 5 in]
        n192 = call <vilib>:"IDtoNode.vi"("error in"=w543, "ID"=w548) -> ("error out"=w544:errorcluster, "invalid Id"=w541:bool, "node ref"=w547:T2)  [unwired: 7 in]
        n193 = call <vilib>:"IDtoNode.vi"("error in"=w544, "ID"=w550) -> ("error out"=w542:errorcluster, "invalid Id"=w540:bool, "node ref"=w549:T2)  [unwired: 7 in]
        n194 = Compound Arithmetic op=AND(w546, invert w541, invert w540) -> (w545:bool)
        n195 = case shown="True" w545 {
          tunnel: w550 -> [_ w576]
          tunnel: w560 -> [_ w578]
          tunnel: [_ TRUE] -> w559
          tunnel: w548 -> [_ w574]
          tunnel: w555 -> [w562 w573]
          tunnel: [w562 w569] -> w553
          tunnel: [w561 w568] -> w552
          tunnel: w549 -> [_ w564]
          tunnel: w547 -> [_ w563]
          tunnel: w542 -> [w561 w565]
          frame False {
          }
          frame True {
            n196 = invoke class="Tree (strict)" method="Edit Tree Items.Move Item"(reference=w578, error in=w565, "tag"=w576, "New Parent"=w574) -> (error out=w566:errorcluster)  [unwired: 3 in, 6 out]
            n197 = Bundle By Name(cluster=T13 {"node ref"=refnum, "new parent"=refnum} ("Cluster"), "new parent"=w563, "node ref"=w564) -> (w572:T13)
            n198 = Flatten To String(anything=w572, error in (no error)=w566) -> (data string=w571:string, error out=w567:errorcluster)  [unwired: 2 in, 1 out]
            n199 = call <vilib>:"Send Local Message.vi"("message queue in"=w573, "message name"="Move", "message value"=w571, "error in"=w567) -> ("message queue out"=w569:T11, "error out"=w568:errorcluster)  [unwired: 9 in, 1 out]
          }
        }
        n200 = event-data("Accepted?"=w559) -> ()  [unwired: 1 in, 1 out]
      }
      event "Exit": Value Change {
        # "Exit the application                                           >> Stop this message generator loop    Cleaning errors if the other loop stop this one"
        n201 = event-data() -> ()  [unwired: 1 in, 1 out]
        n202 = call <vilib>:"Send Local Message.vi"("message queue in"=w583, "message name"="Close", "error in"=w581) -> ("message queue out"=w579:T11, "error out"=w584:errorcluster)  [unwired: 10 in, 1 out]
        n203 = call <vilib>:"Clear Errors.vi"("error in (no error)"=w584) -> ("error out"=w580:errorcluster)  [unwired: 5 in, 1 out]
      }
      event "View": Drag Starting? {
        n204 = event-data() -> ("Data"=w596:T19, "CtlRef"=w598:refnum<vi>, "Coords"=w597:T18)  [unwired: 1 in]
        n205 = invoke class="Tree (strict)" method="Point To Row Column"(reference=w598, error in=w589, "Point"=w597) -> (error out=w588:errorcluster, "Tag"=w595:string)  [unwired: 5 in, 6 out]
        n206 = call <vilib>:"IDtoNode.vi"("error in"=w588, "ID"=w595) -> ("error out"=w587:errorcluster, "invalid Id"=w594:bool, "node ref"=w593:T2)  [unwired: 7 in]
        n207 = case shown="False" w594 {
          tunnel: w593 -> [w606 _]
          tunnel: [w603 TRUE ("Removable")] -> w591
          tunnel: w587 -> [w602 w612]
          tunnel: [w599 w612] -> w586
          frame False {
            n208 = in-place {
              in-place-border: [w609] -> w605
              in-place-border: w602 -> [w608]
              in-place-border: [w607] -> w601
              n209 = in-place-dvr #8(w606) -> (w611:refnum<class "NISE_CEF_Node.lvclass">)  [unwired: 1 out]
              n210 = call-dynamic "EditOptions.vi"("error in"=w608, "node in"=w611) -> ("error out"=w607:errorcluster, "edit options"=w609:T20, "node out"=w610:refnum<class "NISE_CEF_Node.lvclass">)  [unwired: 6 in, 1 out]
              n211 = in-place-dvr #8(w610) -> (w600:errorcluster)  [unwired: 1 out]
            }
            n212 = Unbundle By Name(w605) -> ("movable"=w604:bool)
            n213 = Merge Errors(w600, w601) -> (w599:errorcluster)
            n214 = Not(x=w604) -> (.not. x?=w603:bool)
          }
          frame True {
          }
        }
        n215 = event-data("Data"=w596, "Drag Mode"=enum32{"copy or move", "copy only", "move only"}."move only", "Discard?"=w591) -> ()  [unwired: 1 in, 1 out]
      }
      event "View": Value Change {
        n216 = event-data() -> ("NewVal"=w617:string)  [unwired: 1 in]
        n217 = call <vilib>:"Send Local Message.vi"("message queue in"=w619, "message name"="ActivateNode" ("Message Name"), "message value"=w617, "error in"=w614) -> ("message queue out"=w616:T11, "error out"=w615:errorcluster)  [unwired: 9 in, 1 out]
      }
      event "View": event type 3.0.xa000003a {
        n218 = event-data() -> ("CtlRef"=w628:refnum<vi>, "Coords"=w625:T18)  [unwired: 1 in]
        n219 = invoke class="Tree (strict)" method="Point To Row Column"(reference=w628, error in=w622, "Point"=w625) -> (reference out=w627:refnum<vi>, error out=w621:errorcluster, "Tag"=w626:string)  [unwired: 5 in, 5 out]
        n220 = call <vilib>:"ValidDragDrop.vi"("error in"=w621, "drag over"=w626, "tree ref in"=w627) -> ("error out"=w620:errorcluster, "accepted"=w624:bool)  [unwired: 5 in, 2 out]
        n221 = event-data("Accepted?"=w624) -> ()  [unwired: 1 in, 1 out]
      }
      event Panel Close? {
        # "Intercepts the upper right close panel operation to allow a smooth shutdown as opposed to immediately killing the app."
        n222 = event-data() -> ()  [unwired: 1 in, 1 out]
        n223 = call <vilib>:"Send Local Message.vi"("message queue in"=w633, "message name"="Close?", "error in"=w630) -> ("message queue out"=w631:T11, "error out"=w629:errorcluster)  [unwired: 10 in, 1 out]
        n224 = event-data("Discard?"=TRUE) -> ()  [unwired: 1 in, 1 out]
      }
      event Menu Selection (User) {
        # "#USERCFG It is needed to add a Case for Every item on the menu"
        n225 = event-data() -> ("ItemTag"=w635:string, "ItemPath"=w640:string)  [unwired: 1 in]
        n226 = case shown="Default" w640 {
          selector: w640 -> [w644 _ _ _ _ _ _]
          tunnel: w639 -> [w649 w654 w659 w664 w669 w674 w683]
          tunnel: [w649 w650 w655 w660 w665 w670 w680] -> w638
          tunnel: w637 -> [w646 w652 w657 w662 w667 w672 w679]
          tunnel: [w645 w651 w656 w661 w666 w671 w677] -> w636
          tunnel: w635 -> [w643 _ _ _ _ _ _]
          frame Default {
            n227 = Concatenate Strings(w643, "::" ("string"), w644) -> (w642:string)
            n228 = call <vilib>:"NISE_error generator.vi"("error in"=w646, "source"="configuration tool main.vi", "append error message"=w642, "error code (0)"=538506) -> ("error out"=w645:errorcluster)  [unwired: 5 in]
          }
          frame "_File:_New" {
            n229 = call <vilib>:"Send Local Message.vi"("message queue in"=w654, "message name"="New?" ("Message Name"), "error in"=w652) -> ("message queue out"=w650:T11, "error out"=w651:errorcluster)  [unwired: 10 in, 1 out]
          }
          frame "_File:_Open" {
            n230 = call <vilib>:"Send Local Message.vi"("message queue in"=w659, "message name"="Open?" ("Message Name"), "error in"=w657) -> ("message queue out"=w655:T11, "error out"=w656:errorcluster)  [unwired: 10 in, 1 out]
          }
          frame "_File:_Save" {
            n231 = call <vilib>:"Send Local Message.vi"("message queue in"=w664, "message name"="Save" ("Message Name"), "error in"=w662) -> ("message queue out"=w660:T11, "error out"=w661:errorcluster)  [unwired: 10 in, 1 out]
          }
          frame "_File:Save As..." {
            n232 = call <vilib>:"Send Local Message.vi"("message queue in"=w669, "message name"="SaveAs" ("Message Name"), "error in"=w667) -> ("message queue out"=w665:T11, "error out"=w666:errorcluster)  [unwired: 10 in, 1 out]
          }
          frame "_File:_Exit" {
            n233 = call <vilib>:"Send Local Message.vi"("message queue in"=w674, "message name"="Close?" ("Message Name"), "error in"=w672) -> ("message queue out"=w670:T11, "error out"=w671:errorcluster)  [unwired: 10 in, 1 out]
          }
          frame "_Tools:Multiple Parameter Editor" {
            n234 = call <vilib>:"Send Local Message.vi"("message queue in"=w683, "message name"="CleansubPanel", "error in"=w679) -> ("message queue out"=w682:T11, "error out"=w678:errorcluster)  [unwired: 10 in, 1 out]
            n235 = call <vilib>:"Send Local Message.vi"("message queue in"=w682, "message name"="Custom View" ("Message Name"), "message value"="Multiple Variable Editor" ("Message Name"), "error in"=w678) -> ("message queue out"=w680:T11, "error out"=w677:errorcluster)  [unwired: 9 in, 1 out]
          }
        }
      }
      event User Event {
        n236 = event-data() -> ("node ref"=w684:T2)  [unwired: 1 in]
        n237 = call <vilib>:"NodetoID.vi"("node ref"=w684) -> ("ID"=w687:string)  [unwired: 9 in, 1 out]
        n238 = call <vilib>:"Send Local Message.vi"("message queue in"=w685, "message name"="NodeDataChange", "message value"=w687) -> ("message queue out"=w686:T11)  [unwired: 10 in, 2 out]
      }
    }
    n239 = call "Error.vi"("error in (no error)"=w465, "message queue in"=w466) -> ()  [unwired: 9 in, 1 out]
  }
  n240 = Unregister For Events(event registration refnum=w1) -> (error out=w2:errorcluster)  [unwired: 1 in]
  n241 = Merge Errors(w2, w7) -> (w3:errorcluster)
  n242 = call <vilib>:"DestroyStandardEvents.vi"("error in"=w3, "standard events"=w6) -> ()  [unwired: 9 in, 1 out]
